vi "rotated_picture_init.vi"(11 "Picture FIle Name":string) -> (3 "RotatedPictureInfo":T1)   [LabVIEW 2019]
doc: "Initialize a PNG image to be rotated."
uses:
  Rotated_Picture_TypeDef.ctl
panel:
  out "appended path":path
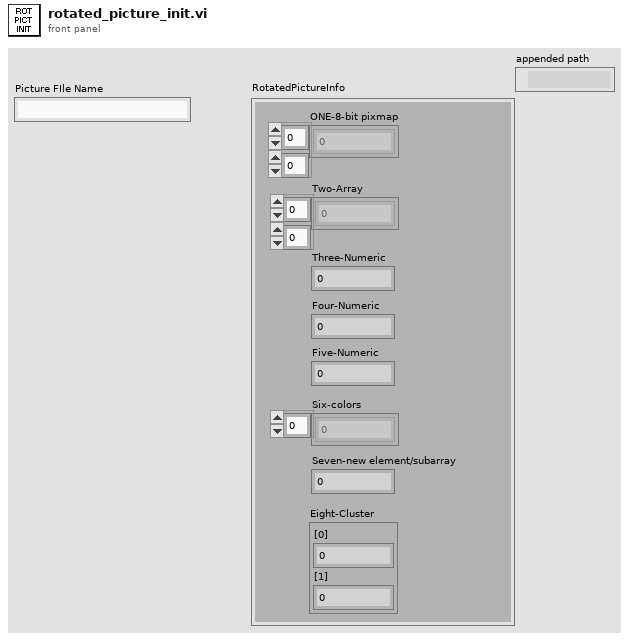
[diagram p1: front panel]
types:
  T1 = typedef "Rotated_Picture_TypeDef.ctl" = cluster{"ONE-8-bit pixmap":u8[][], "Two-Array":cdb[][], "Three-Numeric":i32, "Four-Numeric":i32, "Five-Numeric":cdb, "Six-colors":u32[], "Seven-new element/subarray":u32, "Eight-Cluster":cluster{"[0]":i32, "[1]":i32}}
  T2 = typedef "imagedata.ctl" = cluster{"image type":i32, "image depth":i32, "image":u8[], "mask":u8[], "colors":u32[], "Rectangle":cluster{"left":i16, "top":i16, "right":i16, "bottom":i16}}
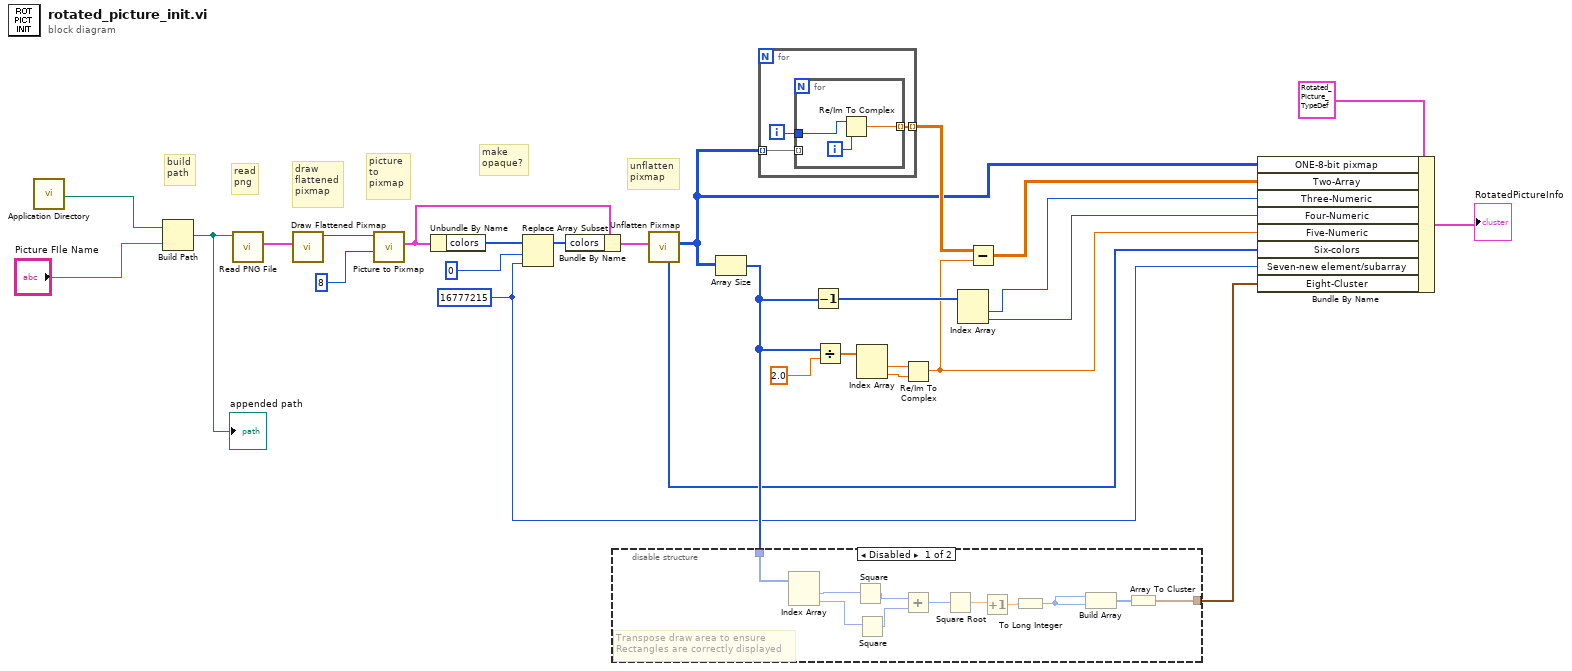
[diagram p0: block diagram]
diagram:
  w4 = u32 16777215 ("new element/subarray")
  # "unflatten\npixmap"
  # "make\nopaque?"
  # "picture\nto\npixmap"
  # "draw\nflattened\npixmap"
  # "read\npng"
  # "build\npath"
  n1 = call <vilib>:"Application Directory.vi"() -> ("Application Directory"=w1:path)
  n2 = Build Path(base path=w1, name or relative path="Picture FIle Name") -> (appended path=w18:path)
  "appended path" <- w18
  n3 = call <vilib>:"Read PNG File.vi"("path to PNG file"=w18) -> ("image data"=w24:T2)  [unwired: 8 in, 2 out]
  n4 = call <vilib>:"Draw Flattened Pixmap.vi"("image data"=w24) -> ("new picture"=w25:picture)  [unwired: 8 in]
  n5 = call <vilib>:"Picture to Pixmap.vi"("depth"=8, "picture"=w25) -> ("image data"=w27:T2)  [unwired: 8 in, 1 out]
  n6 = Unbundle By Name(w27) -> ("colors"=w21:u32[])
  n7 = Replace Array Subset(array=w21, new element=w4, index=0) -> (w23:u32[])
  n8 = Bundle By Name(cluster=w27, "colors"=w23) -> (w28:T2)
  n9 = call <vilib>:"Unflatten Pixmap.vi"("image data"=w28) -> ("8-bit pixmap"=w10:u8[][], "colors"=w5:u32[])  [unwired: 4 in, 5 out]
  n10 = Array Size(array=w10) -> (size(s)=w20:i32[])
  n11 = disable-structure shown="Disabled" {
    disable-tunnel: w20 -> [w39 _]
    disable-tunnel: [w29 _] -> w3
    frame Disabled {
      # "Transpose draw area to ensure \nRectangles are correctly displayed"
      n12 = Index Array(array=w39) -> (element #1=w38:i32, element #2=w37:i32)  [unwired: 2 in]
      n13 = Square(x=w38) -> (x^2=w36:i32)
      n14 = Square(x=w37) -> (x^2=w35:i32)
      n15 = Add(x=w36, y=w35) -> (x+y=w34:i32)
      n16 = Square Root(x=w34) -> (sqrt(x)=w33:dbl)
      n17 = Increment(x=w33) -> (x+1=w32:dbl)
      n18 = To Long Integer(number=w32) -> (32bit integer=w31:i32)
      n19 = Build Array(w31, w31) -> (w30:i32[])
      n20 = Array To Cluster(array=w30) -> (cluster=w29:cluster{"[0]":i32, "[1]":i32})
    }
    frame Enabled {
    }
  }
  n21 = for {
    tunnel: [w41] -> w12 mode=indexing
    tunnel: w10 -> [w40] mode=indexing
    i -> [w42]
    n22 = for {
      tunnel: w42 -> [w45]
      tunnel: [w44] -> w41 mode=indexing
      tunnel: w40 -> [_] mode=indexing
      i -> [w43]
      n23 = Re/Im To Complex(1:w43, 2:w45) -> (0:w44:cdb)
    }
  }
  n24 = Decrement(x=w20) -> (x-1=w17:i32[])
  n25 = Divide(x=w20, y=2.0) -> (x/y=w14:dbl[])
  n26 = Index Array(array=w14) -> (element #1=w15:dbl, element #2=w16:dbl)  [unwired: 2 in]
  n27 = Re/Im To Complex(1:w16, 2:w15) -> (0:w6:cdb)
  n28 = Index Array(array=w17) -> (element #1=w8:i32, element #2=w7:i32)  [unwired: 2 in]
  n29 = Subtract(x=w12, y=w6) -> (x-y=w9:cdb[][])
  n30 = Bundle By Name(cluster=T1 {"ONE-8-bit pixmap"=[], "Two-Array"=[], "Three-Numeric"=0, "Four-Numeric"=0, "Five-Numeric"=0.0+0.0i, "Six-colors"=[], "Seven-new element/subarray"=0, "Eight-Cluster"={"[0]"=0, "[1]"=0}} ("RotatedPictureInfo"), "ONE-8-bit pixmap"=w10, "Two-Array"=w9, "Three-Numeric"=w8, "Four-Numeric"=w7, "Five-Numeric"=w6, "Six-colors"=w5, "Seven-new element/subarray"=w4, "Eight-Cluster"=w3) -> (→"RotatedPictureInfo":T1)
